vi "Create New File.vi"(8 "error in (no error)":errorcluster, 11 "Logger in":refnum<class "Logger.lvclass">) -> (0 "error out":errorcluster, 3 "Logger out":refnum<class "Logger.lvclass">)   [LabVIEW 2017, in "Logger.lvlib" / "Logger.lvclass"]
uses:
  Logger.lvclass
  Logger.lvclass/Logger.ctl
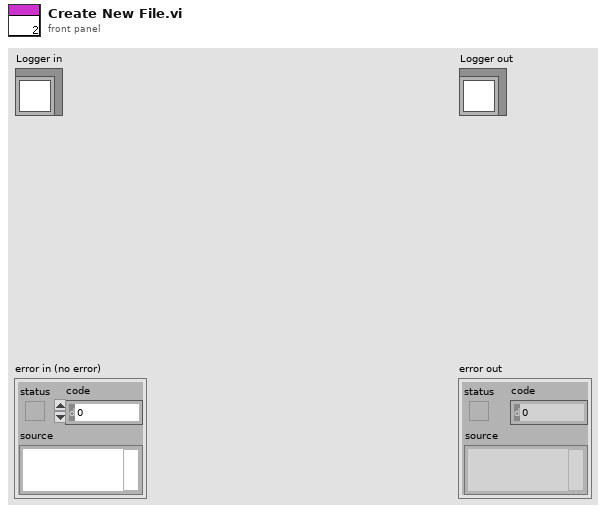
[diagram p1: front panel]
types:
  T1 = enum16{"open", "open or create", "create or replace", "create", "open (read-only)"}
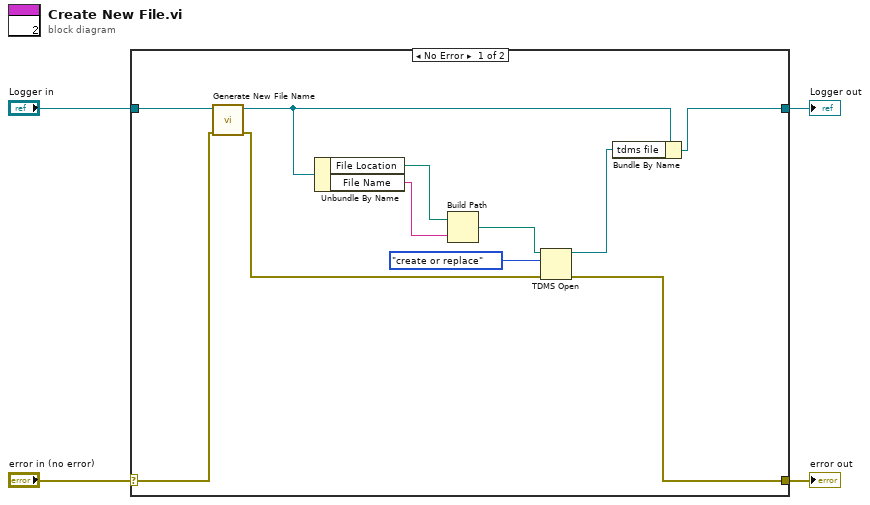
[diagram p0: block diagram]
diagram:
  n1 = case shown="No Error" "error in (no error)" {
    selector: "error in (no error)" -> [w6 w17]
    tunnel: [w5 w17] -> w3
    tunnel: [w8 w16] -> w1
    tunnel: "Logger in" -> [w15 w16]
    frame No Error {
      n2 = call-dynamic "Generate New File Name.vi"("error in (no error)"=w6, "Logger in"=w15) -> ("error out"=w7:errorcluster, "Logger out"=w10:refnum<class "Logger.lvclass">)  [unwired: 8 in]
      n3 = Unbundle By Name(w10) -> ("File Location"=w14:path, "File Name"=w13:string)
      n4 = Build Path(base path=w14, name or relative path=w13) -> (appended path=w12:path)
      n5 = TDMS Open(8:w7, 10:T1."create or replace" ("operation (0:open)"), 11:w12) -> (0:w5:errorcluster, 3:w9:refnum<k34>)  [unwired: 4 in]
      n6 = Bundle By Name(cluster=w10, "tdms file"=w9) -> (w8:refnum<class "Logger.lvclass">)
    }
    frame Error {
    }
  }
  "error out" <- w3
  "Logger out" <- w1
